vi "Get Port Properties.vi"(8 "Error In":errorcluster, 11 "Device Name":string="Basys2") -> (0 "Error Out":errorcluster, 2 "Port Properties":T1, 3 "HIF":u32)   [LabVIEW 2011, in "LVH-Adept.lvlib"]
uses:
  LVH-Adept.lvlib
  Private/DJTG/Private/Type Defs/Port Properties.ctl
  Private/DMGR/DMGR.lvlib
  Private/DJTG/DJTG.lvlib
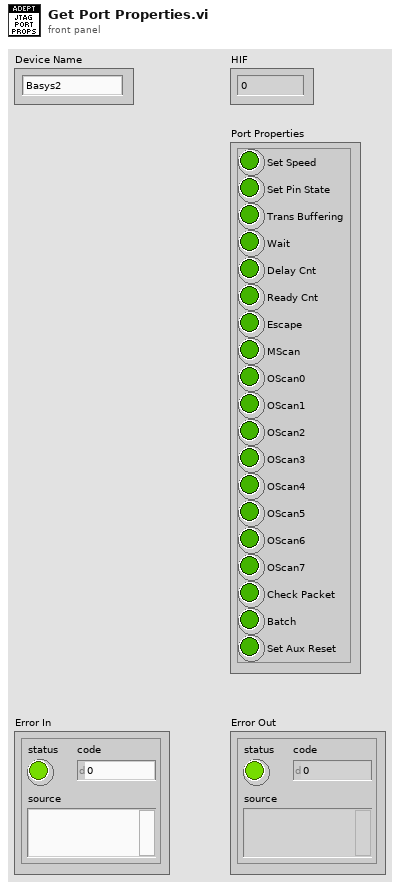
[diagram p1: front panel]
types:
  T1 = typedef "LVH-Adept.lvlib/DJTG.lvlib/Port Properties.ctl" = cluster{"Set Speed":bool, "Set Pin State":bool, "Trans Buffering":bool, "Wait":bool, "Delay Cnt":bool, "Ready Cnt":bool, "Escape":bool, "MScan":bool, "OScan0":bool, "OScan1":bool, "OScan2":bool, "OScan3":bool, "OScan4":bool, "OScan5":bool, "OScan6":bool, "OScan7":bool, "Check Packet":bool, "Batch":bool, "Set Aux Reset":bool}
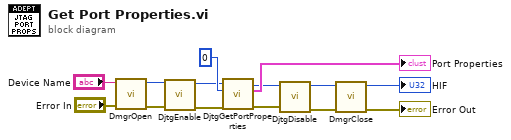
[diagram p0: block diagram]
diagram:
  n1 = call "DmgrOpen.vi"("Error In"="Error In", "Device Name"="Device Name") -> ("Error Out"=w8:errorcluster, "Device Handle"=w9:u32)  [unwired: 8 in]
  n2 = call "DjtgEnable.vi"("Error In"=w8, "Device Number"=w9) -> ("Error Out"=w7:errorcluster, "Device Number"=w6:u32)  [unwired: 8 in]
  n3 = call "DjtgGetPortProperties.vi"("Error In"=w7, "Port Number"=0, "Device Number"=w6) -> ("Error Out"=w5:errorcluster, "Port Properties"=→"Port Properties":T1, "Device Number"=w2:u32)  [unwired: 6 in]
  n4 = call "DjtgDisable.vi"("Error In"=w5, "Device Number"=w2) -> ("Error Out"=w4:errorcluster, "Device Number"=w3:u32)  [unwired: 8 in]
  "HIF" <- w3
  n5 = call "DmgrClose.vi"("Error In"=w4, "hif"=w3) -> ("Error Out"=→"Error Out":errorcluster)  [unwired: 9 in]
